vi "UDP Data Link - Configuration Utilities - Set Tx Remove Channel Button.vi"(8 "error in (no error)":errorcluster, 11 "Tx ItemNames":string[][](array[string])) -> (0 "error out":errorcluster)   [LabVIEW 2015, in "UDP Data Link System Explorer.lvlib"]
uses:
  UDP Data Link System Explorer.lvlib
  Shared/UDP Data Link Global.vi
  <vilib>/NI Veristand/Custom Device API/Custom Device API.lvlib
  Shared/UDP Data Link Shared.lvlib
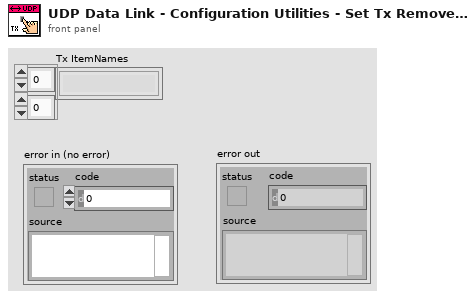
[diagram p1: front panel]
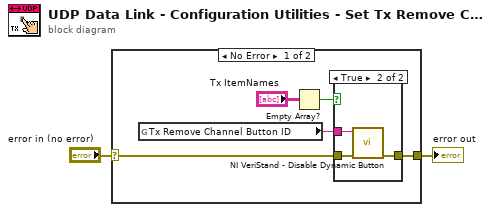
[diagram p0: block diagram]
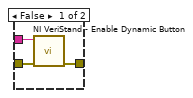
[diagram p2: hidden frame]
diagram:
  n1 = case shown="No Error" "error in (no error)" {
    selector: "error in (no error)" -> [w4 w14]
    tunnel: [w3 w14] -> w1
    frame No Error {
      n2 = global read "UDP Data Link Global.vi" "Tx Remove Channel Button ID"() -> (w7:string)
      n3 = Empty Array?(array="Tx ItemNames") -> (empty?=w6:bool)
      n4 = case shown="True" w6 {
        tunnel: w7 -> [w10 w13]
        tunnel: w4 -> [w9 w12]
        tunnel: [w8 w11] -> w3
        frame False {
          n5 = call <vilib>:"NI VeriStand - Enable Dynamic Button.vi"("error in (no error)"=w9, "Button ID"=w10) -> ("error out"=w8:errorcluster)  [unwired: 9 in]
        }
        frame True {
          n6 = call <vilib>:"NI VeriStand - Disable Dynamic Button.vi"("error in (no error)"=w12, "Button ID"=w13) -> ("error out"=w11:errorcluster)  [unwired: 9 in]
        }
      }
    }
    frame Error {
    }
  }
  "error out" <- w1
